vi "_Buffer_RefError.vi"(10 "error in (no error)":errorcluster) -> (2 "error out":errorcluster)   [LabVIEW 2013, in "CircularBuffer.lvlib" / "VariantBuffer.lvclass"]
uses:
  VariantBuffer.lvclass
  buffer-errors -- ring.ctl
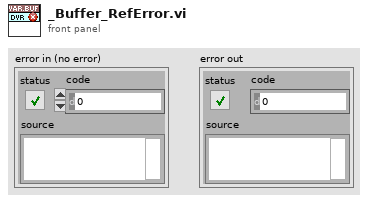
[diagram p1: front panel]
types:
  T1 = typedef "CircularBuffer.lvlib/VariantBuffer.lvclass/buffer-errors -- ring.ctl" = i32
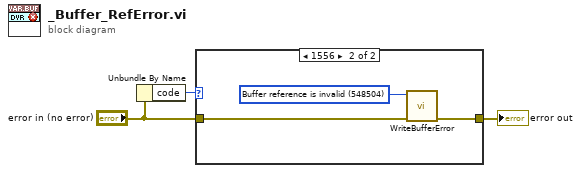
[diagram p0: block diagram]
diagram:
  n1 = Unbundle By Name("error in (no error)") -> ("code"=w1:i32)
  n2 = case shown="1556" w1 {
    tunnel: [w4 w7] -> w3
    tunnel: "error in (no error)" -> [w4 w6]
    frame Default {
    }
    frame 1556 {
      w5 = T1 548504 items=["No error"=0, "Generic Buffer error"=548500, "Buffer is full"=548501, "Buffer is empty"=548502, "Buffer size cannot be 0"=548503, "Buffer reference is invalid"=548504, "Buffer event reference invalid"=548505, "Buffer Type not supported"=548506, "Not enough space in the buffer for this operation"=548507] ("buffer-errors")
      n3 = call "WriteBufferError.vi"("error in (no error)"=w6, "buffer-errors"=w5) -> ("error out"=w7:errorcluster)  [unwired: 9 in]
    }
  }
  "error out" <- w3
